vi "Read Status.vi"(11 "Method Result In":T2={"Test Case"="", "Test Method Name"="", "Status"=enum."Passed", "Assertion Results"=[], "Execution time"=0.0, "Result String"=""}) -> (1 "Glyph Index":i32=5, 2 "Status":T1, 3 "Method Result Out":T2={"Test Case"="", "Test Method Name"="", "Status"=enum."Passed", "Assertion Results"=[], "Execution time"=0.0, "Result String"=""})   [LabVIEW 2020, in "Method Result.lvlib"]
uses:
  Method Result.lvlib
  Method Result.ctl
  Core/Result/Status.ctl
  Assertion Result/Assertion Result.ctl
  Assertion Result/Public/TypeDefs/Assertion Type.ctl
  Assertion Result/Public/TypeDefs/Status.ctl
  Assertion Result/Assertion Result.lvlib
  Core/Result/Result.lvlib
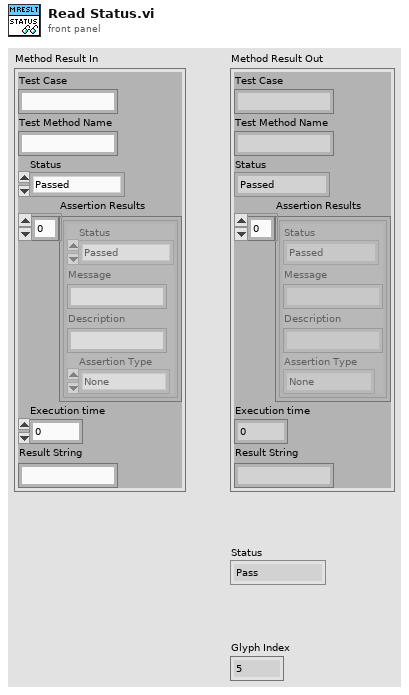
[diagram p1: front panel]
types:
  T1 = typedef "Assertion Result.lvlib/Status.ctl" = enum16{"Pass", "Fail", "Error", "Skipped", "Setup Error", "Broken", "Teardown Error"}
  T2 = typedef "Method Result.lvlib/Method Result.ctl" = cluster{"Test Case":string, "Test Method Name":string, "Status":T3, "Assertion Results":T4[], "Execution time":dbl, "Result String":string}
  T3 = typedef "Result.lvlib/Status.ctl" = enum16{"", "Passed", "Failed", "Error", "Skipped", "Setup Error", "Broken", "Teardown Error"}
  T4 = typedef "Assertion Result.lvlib/Assertion Result.ctl" = cluster{"Status":T3, "Message":string, "Description":string, "Assertion Type":T5}
  T5 = typedef "Result.lvlib/Assertion Type.ctl" = enum16{"None", "Pass", "Fail", "Skip", "Pass if Equal", "Fail if Equal", "Pass if Error", "Fail if Error", "Pass if", "Fail if"}
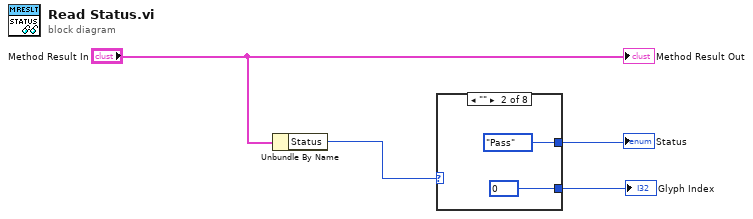
[diagram p0: block diagram]
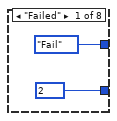
[diagram p2: hidden frame]
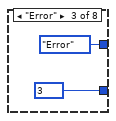
[diagram p3: hidden frame]
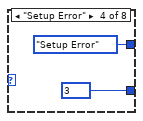
[diagram p4: hidden frame]
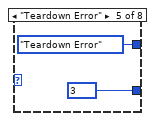
[diagram p5: hidden frame]
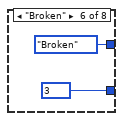
[diagram p6: hidden frame]
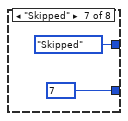
[diagram p7: hidden frame]
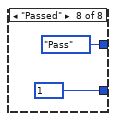
[diagram p8: hidden frame]
diagram:
  n1 = Unbundle By Name("Method Result In") -> ("Status"=w2:T3)
  n2 = case shown="\"\"" w2 {
    tunnel: [2 ("Listbox Symbol Ring Constant") 0 ("Listbox Symbol Ring Constant") 3 ("Listbox Symbol Ring Constant") 3 ("Listbox Symbol Ring Constant") 3 ("Listbox Symbol Ring Constant") 3 ("Listbox Symbol Ring Constant") 7 ("Listbox Symbol Ring Constant") 1 ("Listbox Symbol Ring Constant")] -> w3
    tunnel: [Status."Fail" ("Status") Status."Pass" ("Status") Status."Error" ("Status") Status."Setup Error" ("Status") Status."Teardown Error" ("Status") Status."Broken" ("Status") Status."Skipped" ("Status") Status."Pass" ("Status")] -> w1
    frame "Failed" {
    }
    frame "" {
    }
    frame "Error" {
    }
    frame "Setup Error" {
    }
    frame "Teardown Error" {
    }
    frame "Broken" {
    }
    frame "Skipped" {
    }
    frame "Passed" {
    }
  }
  "Status" <- w1
  "Glyph Index" <- w3
  "Method Result Out" <- "Method Result In"
